vi "TcA04-004_NestedObjectsCallsDynamicMethods.vi"(1 "Input buffer":T3="1", 3 "Invocation info":T2, 5 "error in (no error)":errorcluster, 6 "Add log to result?":bool) -> (16 "Test Data":T1 {"Numeric Measurement" format="%.2f"}, 19 "error out":errorcluster)   [LabVIEW 2009]
doc: "Test case template."
uses:
  Shared/Support_InputBuffer.ctl
  Shared/Support_InvocationInfo.ctl
  Shared/Support_TestData.ctl
  TestClasses/G#BaseClass1_class/G#BaseClass1.lvclass
  TestClasses/G#SubSubClass1_class/G#SubSubClass1.lvclass
  TestClasses/G#SubClass1_class/G#SubClass1.lvclass
  <vilib>/addons/_AddQ/G#Object/G#Object.lvclass
panel:
  in  "Test name":string="TcA04-004 Nested objects calls dynamic methods"
  out "Test result":bool
  out "Result":string
  # "Verify that an object from a different class can\ndynamically call a virtual declared base class method."
  # "Sub test case"
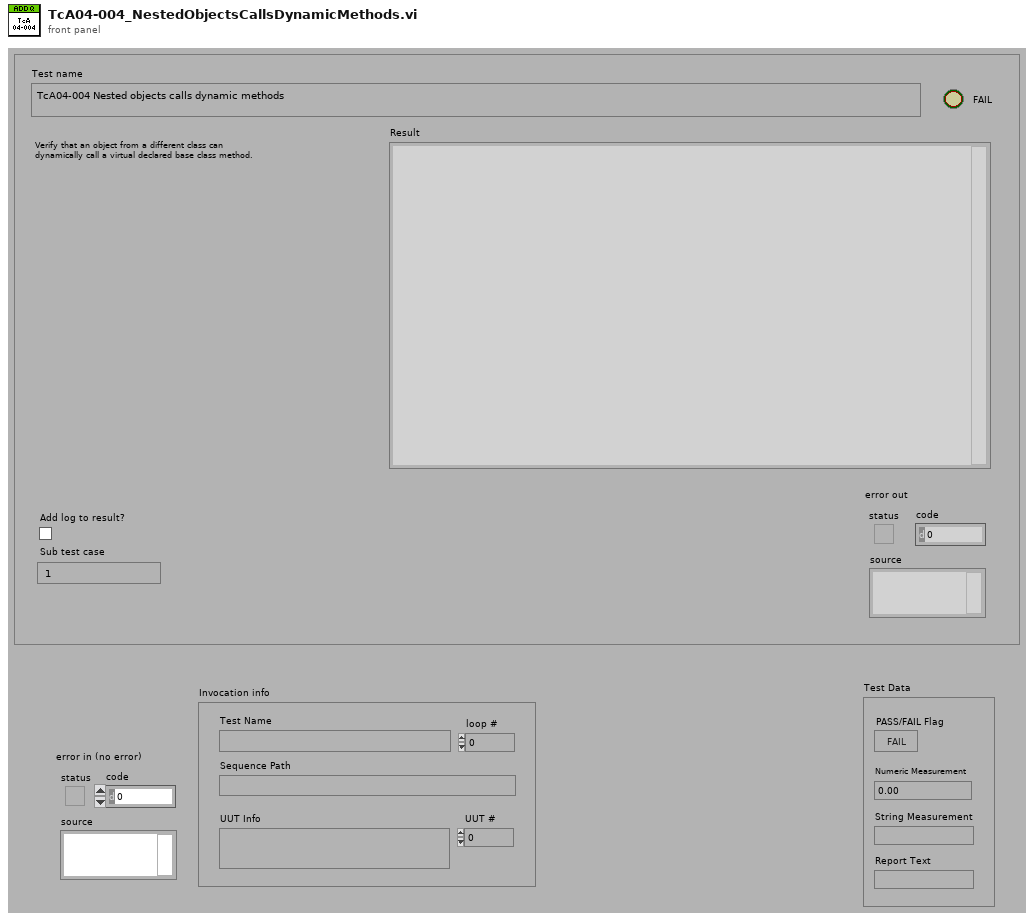
[diagram p1: front panel]
types:
  T1 = typedef "Support_TestData.ctl" = cluster{"PASS/FAIL Flag":bool, "Numeric Measurement":dbl, "String Measurement":string, "Report Text":string}
  T2 = typedef "Support_InvocationInfo.ctl" = cluster{"UUT #":i32, "loop #":i32, "UUT Info":string, "Test Name":string, "Sequence Path":path}
  T3 = typedef "Support_InputBuffer.ctl" = string
  T4 = typedef "Support_ResultType.ctl" = cluster{"Pass":bool, "Comment":string, "MeasurementValue":dbl}
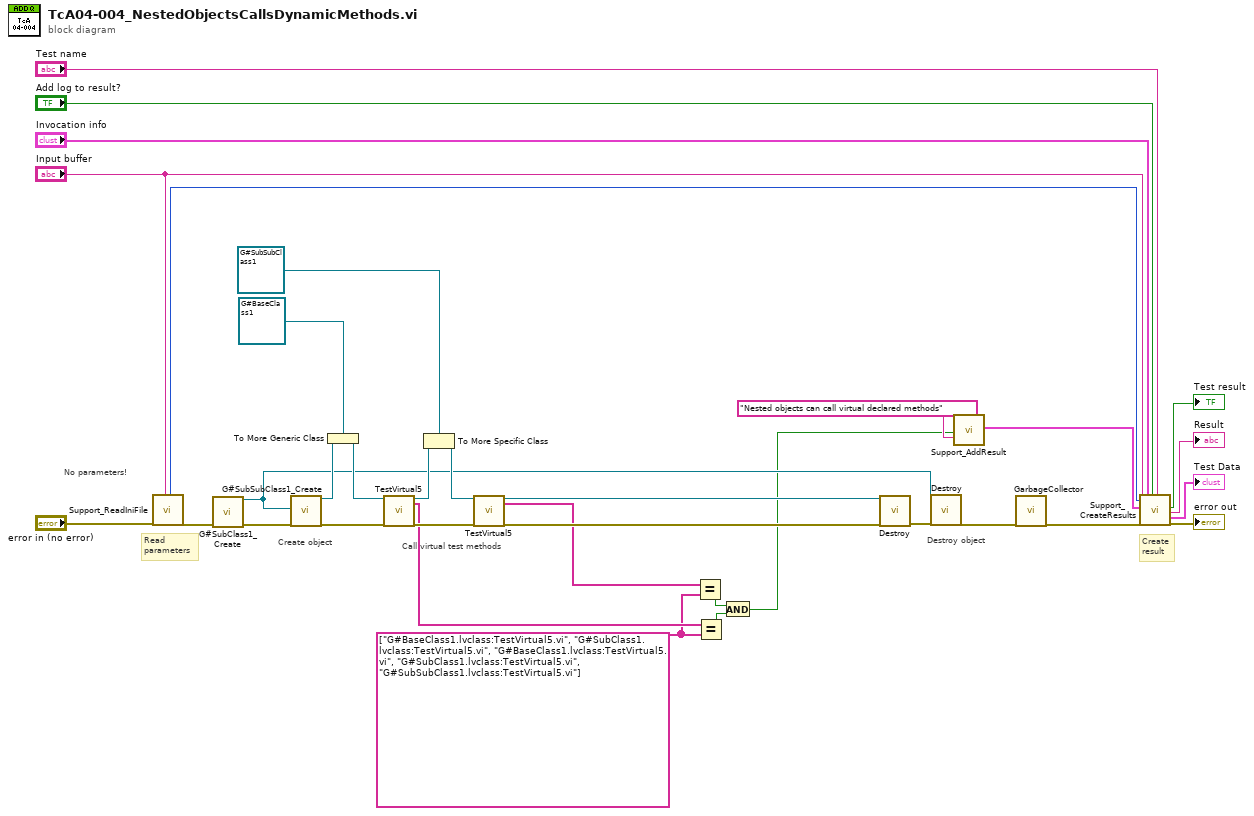
[diagram p0: block diagram]
diagram:
  w5 = string[] ["G#BaseClass1.lvclass:TestVirtual5.vi", "G#SubClass1.lvclass:TestVirtual5.vi", "G#BaseClass1.lvclass:TestVirtual5.vi", "G#SubClass1.lvclass:TestVirtual5.vi", "G#SubSubClass1.lvclass:TestVirtual5.vi"] ("MethodName")
  # "Destroy object"
  # "Call virtual test methods"
  # "Create object"
  # "No parameters!"
  # "Create\nresult"
  # "Read\nparameters"
  n1 = call "Support_ReadIniFile.vi"("error in (no error)"="error in (no error)", "Sub test case"="Input buffer") -> ("Timer start"=w24:u32, "error out"=w11:errorcluster)  [unwired: 10 in, 6 out]
  n2 = call "G#SubClass1_Create.vi"("error in (no error)"=w11) -> ("reference out"=w9:refnum<class "G#SubClass1.lvclass">, "error out"=w10:errorcluster)  [unwired: 16 in, 1 out]
  n3 = call "G#SubSubClass1_Create.vi"("G#BaseClass1.lvclass"=w9, "error in (no error)"=w10) -> ("reference out"=w19:refnum<class "G#SubSubClass1.lvclass">, "error out"=w23:errorcluster)  [unwired: 16 in]
  n4 = To More Generic Class(target class=refnum<class "G#BaseClass1.lvclass"> refnum ("G#BaseClass1.lvclass"), reference=w19) -> (generic class reference=w18:refnum<class "G#BaseClass1.lvclass">)
  n5 = call-dynamic "TestVirtual5.vi"("reference in"=w18, "error in (no error)"=w23) -> ("reference out"=w17:refnum<class "G#BaseClass1.lvclass">, "MethodName"=w6:string[], "error out"=w22:errorcluster)  [unwired: 15 in]
  n6 = To More Specific Class(target class=refnum<class "G#SubSubClass1.lvclass"> refnum ("G#SubSubClass1.lvclass"), reference=w17) -> (specific class reference=w16:refnum<class "G#SubSubClass1.lvclass">)  [unwired: 1 in, 1 out]
  n7 = call-dynamic "TestVirtual5.vi"("reference in"=w16, "error in (no error)"=w22) -> ("reference out"=w7:refnum<class "G#SubSubClass1.lvclass">, "MethodName"=w4:string[], "error out"=w8:errorcluster)  [unwired: 15 in]
  n8 = Equal?(x=w4, y=w5) -> (x = y?=w3:bool)
  n9 = Equal?(x=w6, y=w5) -> (x = y?=w2:bool)
  n10 = And(x=w3, y=w2) -> (x .and. y?=w1:bool)
  n11 = call-dynamic "Destroy.vi"("reference in"=w7, "error in (no error)"=w8) -> ("error out"=w13:errorcluster)  [unwired: 16 in, 1 out]
  n12 = call-dynamic "Destroy.vi"("reference in"=w9, "error in (no error)"=w13) -> ("error out"=w12:errorcluster)  [unwired: 16 in, 1 out]
  n13 = call "Support_AddResult.vi"("Pass"=w1, "Comment"="Nested objects can call virtual declared methods") -> ("Results out"=w27:T4[])  [unwired: 17 in]
  n14 = call <vilib>:"GarbageCollector.vi"("error in (no error)"=w12) -> ("error out"=w21:errorcluster)  [unwired: 16 in, 2 out]
  n15 = call "Support_CreateResults.vi"("Sub test case"="Input buffer", "Timer start"=w24, "Results"=w27, "error in (no error)"=w21, "Invocation info"="Invocation info", "Add log to result?"="Add log to result?", "Test name"="Test name") -> ("Pass/fail flag"=→"Test result":bool, "Result"=→"Result":string, "Test Data"=→"Test Data":T1, "error out"=→"error out":errorcluster)  [unwired: 9 in]
